vi "Create.vi"(8 "error in (no error)":errorcluster, 9 "Config Hash":string, 10 "Config Version":string) -> (0 "error out":errorcluster, 3 "Config Alert Module out":refnum<class "Config Alert Module.lvclass">)   [LabVIEW 2020, in "Volatus.lvlib" / "Config Alert Module.lvclass"]
uses:
  Config Alert Module.lvclass
  Config Alert Module.lvclass/Config Alert Module.ctl
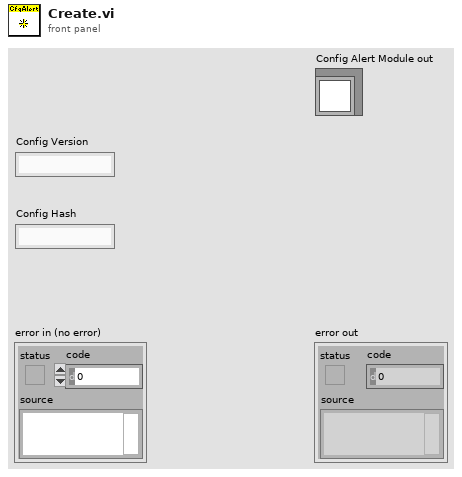
[diagram p1: front panel]
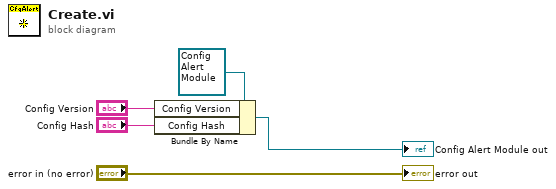
[diagram p0: block diagram]
diagram:
  n1 = Bundle By Name(cluster=refnum<class "Config Alert Module.lvclass"> refnum ("Config Alert Module in"), "Config Version"="Config Version", "Config Hash"="Config Hash") -> (→"Config Alert Module out":refnum<class "Config Alert Module.lvclass">)
  "error out" <- "error in (no error)"
